vi "Replace if Empty.vi"(7 "if empty":string, 10 "Text in":string) -> (2 "Text out":string)   [LabVIEW 2020, in "Approval Tests.lvlib"]
uses:
  Approval Tests.lvlib
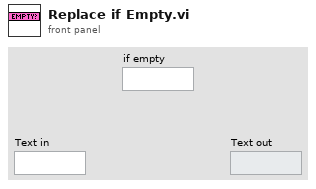
[diagram p1: front panel]
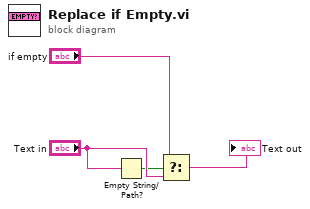
[diagram p0: block diagram]
diagram:
  n1 = Empty String/Path?(string/path="Text in") -> (empty?=w1:bool)
  n2 = Select(t="if empty", s=w1, f="Text in") -> (s? t:f=→"Text out":string)
